vi "Get Configuration.vi"(8 "error in (no error)":errorcluster, 11 "User Interface in":refnum<class "User Interface.lvclass">) -> (0 "error out":errorcluster, 2 "configuration":refnum<class "Configuration.lvclass">, 3 "User Interface out":refnum<class "User Interface.lvclass">)   [LabVIEW 2020, in "DSF Core.lvlib" / "User Interface.lvclass"]
uses:
  User Interface.lvclass
  Configuration/Configuration.lvclass
  User Interface.lvclass/User Interface.ctl
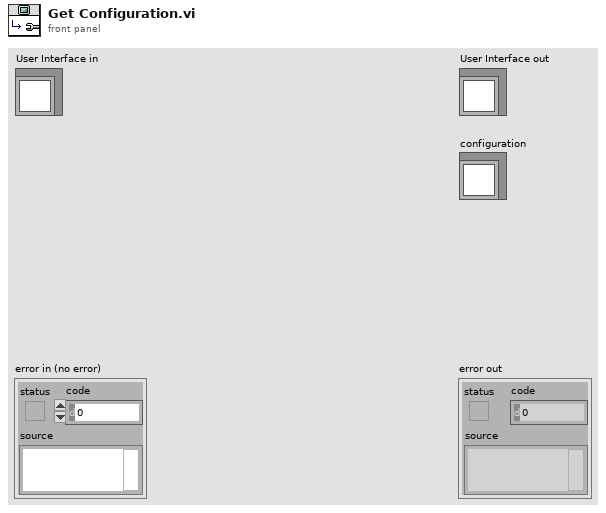
[diagram p1: front panel]
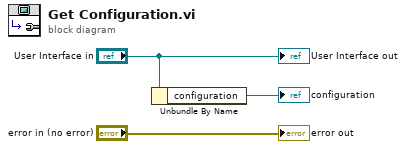
[diagram p0: block diagram]
diagram:
  n1 = Unbundle By Name("User Interface in") -> ("configuration"=→"configuration":refnum<class "Configuration.lvclass">)
  "error out" <- "error in (no error)"
  "User Interface out" <- "User Interface in"
